vi "TTA_Draw_Labelled_Line.vi"(4 "Line Type":T1={"Width"=1, "Style"=enum."Solid"}, 5 "End Point":cluster{"x":i16, "y":i16}, 6 "Line color":u32(colorbox), 7 "Start Point":cluster{"x":i16, "y":i16}, 8 "error in":errorcluster, 9 "Label\nEnd Point":string, 10 "Label\nStart Point":string, 11 "picture":picture) -> (0 "error out":errorcluster, 3 "2D Picture\nOut":picture)   [LabVIEW 2016]
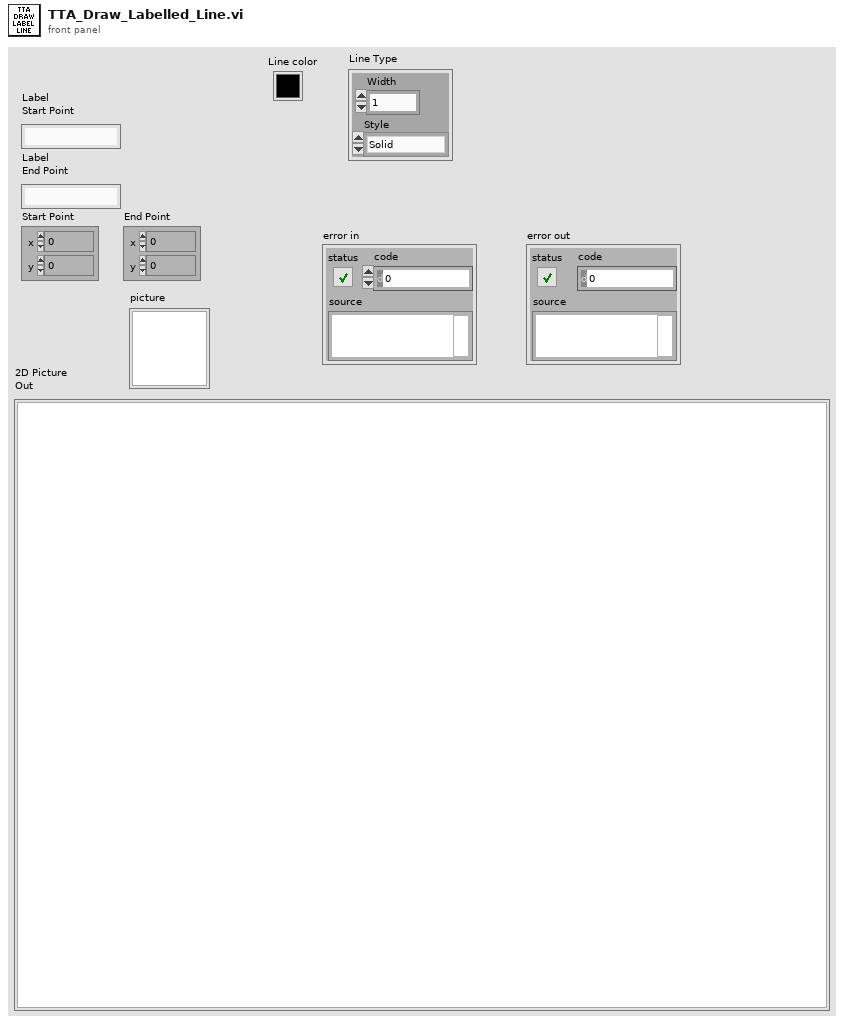
[diagram p1: front panel]
types:
  T1 = cluster{"Width":u16, "Style":enum32{"Solid", "Dash", "Dot", "DashDot", "DashDotDot"}}
  T2 = enum16{"User-specified Font", "Application Font", "System Font", "Dialog Font"}
  T3 = cluster{"Font Name:":string, "Size":i16, "Strikeout?":bool, "Italic?":bool, "Underline?":bool, "Outline?":bool, "Shadow?":bool, "Bold?":bool}
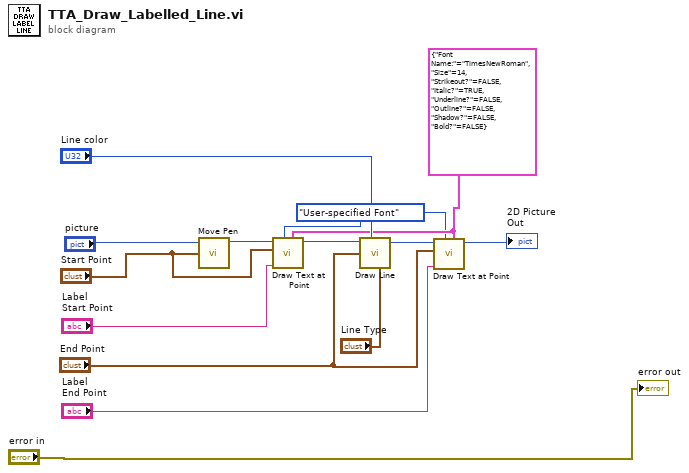
[diagram p0: block diagram]
diagram:
  w1 = T2."User-specified Font" ("desired font(Application)")
  w2 = T3 {"Font Name:"="TimesNewRoman", "Size"=14, "Strikeout?"=FALSE, "Italic?"=TRUE, "Underline?"=FALSE, "Outline?"=FALSE, "Shadow?"=FALSE, "Bold?"=FALSE} ("[user-specified font]")
  n1 = call <vilib>:"Move Pen.vi"("new position"="Start Point", "picture"="picture") -> ("new picture"=w10:picture)  [unwired: 3 in]
  n2 = call <vilib>:"Draw Text at Point.vi"("[user-specified font]"=w2, "desired font(Application)"=w1, "text"="Label\nStart Point", "origin"="Start Point", "picture"=w10) -> ("new picture"=w9:picture)  [unwired: 5 in, 1 out]
  n3 = call <vilib>:"Draw Line.vi"("picture"=w9, "end point"="End Point", "color(black)"="Line color", "pen"="Line Type") -> ("new picture"=w6:picture)  [unwired: 5 in]
  n4 = call <vilib>:"Draw Text at Point.vi"("[user-specified font]"=w2, "desired font(Application)"=w1, "text"="Label\nEnd Point", "origin"="End Point", "picture"=w6) -> ("new picture"=→"2D Picture\nOut":picture)  [unwired: 5 in, 1 out]
  "error out" <- "error in"
